vi "test_filefolder_check.vi"() -> ()   [LabVIEW 2019]
panel:
  out "file or folder exists?":bool caption="파일 또는 폴더가 존재합니까?"
  out "cancelled":bool
  out "dup path":path
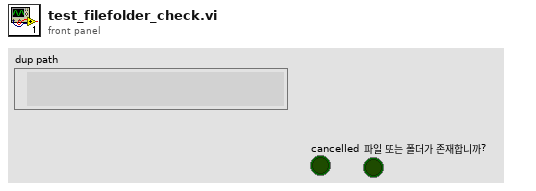
[diagram p1: front panel]
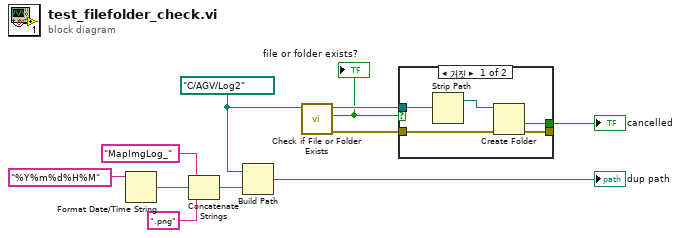
[diagram p0: block diagram]
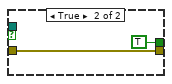
[diagram p2: hidden frame]
diagram:
  w2 = path "C:/AGV/Log2" ("베이스 경로")
  n1 = Format Date/Time String(time format string (%c)="%Y%m%d%H%M") -> (date/time string=w8:string)  [unwired: 2 in]
  n2 = Concatenate Strings("MapImgLog_", w8, ".png" ("문자열")) -> (w4:string)
  n3 = Build Path(base path=w2, name or relative path=w4) -> (appended path=→"dup path":path)
  n4 = call <vilib>:"Check if File or Folder Exists.vi"("path"=w2) -> ("error out"=w5:errorcluster, "file or folder exists?"=w6:bool, "dup path"=w7:path)  [unwired: 8 in]
  "file or folder exists?" <- w6
  n5 = case shown="거짓" w6 {
    tunnel: w7 -> [w16 _]
    tunnel: w5 -> [w15 w18]
    tunnel: [w14 w18] -> _
    tunnel: [w13 TRUE ("cancelled")] -> w3
    frame False {
      n6 = Strip Path(path=w16) -> (stripped path=w12:path)  [unwired: 1 out]
      n7 = Create Folder(path (use dialog)=w12, error in=w15) -> (cancelled=w13:bool, error out=w14:errorcluster)  [unwired: 1 in, 1 out]
    }
    frame True {
    }
  }
  "cancelled" <- w3
